vi "m1m3_logEvent_SettingsApplied.vi"(8 "error in (no error)":errorcluster, 11 "logevent_SettingsApplied_Ctl":T1={"Timestamp"=0.0, "Settings"="                                                                                                                                                                                                                                                                ", "priority"=0}) -> (0 "error out":errorcluster, 2 "function return":i32, 3 "logevent_SettingsApplied_Ctl out":T1={"Timestamp"=0.0, "Settings"="                                                                                                                                                                                                                                                                ", "priority"=0})   [LabVIEW 2016, in "SALLV_m1m3.lvlib"]
doc: "int m1m3_shm_logEvent_SettingsAppliedLV(m1m3_logevent_SettingsAppliedLV *logevent_SettingsApplied_Ctl );"
uses:
  SALLV_m1m3.lvlib
  DataTypes/logevent_SettingsApplied.ctl
  SALLV_m1m3.so
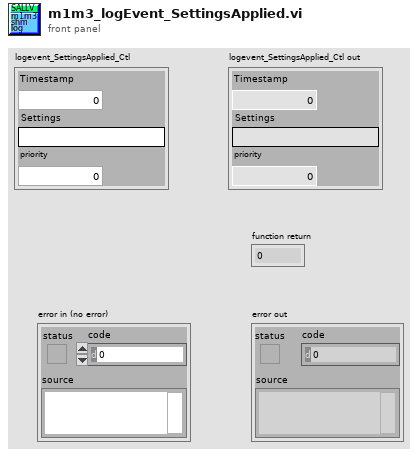
[diagram p1: front panel]
types:
  T1 = typedef "SALLV_m1m3.lvlib/logevent_SettingsApplied.ctl" = cluster{"Timestamp":dbl, "Settings":string, "priority":i32}
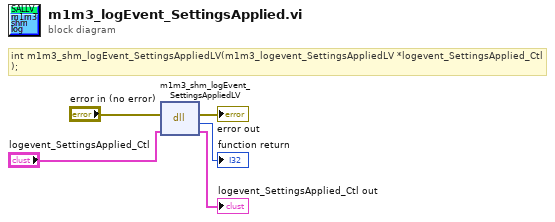
[diagram p0: block diagram]
diagram:
  # "int m1m3_shm_logEvent_SettingsAppliedLV(m1m3_logevent_SettingsAppliedLV *logevent_SettingsApplied_Ctl );"
  n1 = dll-call lib="opt/CODE/SALLV_m1m3/SALLV_m1m3.*" fn="m1m3_shm_logEvent_SettingsAppliedLV"(error in="error in (no error)", "logevent_SettingsApplied_Ctl"="logevent_SettingsApplied_Ctl") -> (error out=→"error out":errorcluster, →"function return":i32, "logevent_SettingsApplied_Ctl"=→"logevent_SettingsApplied_Ctl out":T1)  [unwired: 2 in, 1 out]
